vi "Pass.vi"(8 "error in (no error)":errorcluster, 11 "Constraint in":refnum<class "Constraint.lvclass">) -> (0 "error out":errorcluster, 3 "Constraint out":refnum<class "Constraint.lvclass">)   [LabVIEW 2017, in "Transparent Assertions.lvlib" / "Constraints.lvlib" / "Constraint.lvclass"]
doc: "Reports a successful test."
uses:
  Constraint.lvclass
  Frameworks/Test Framework/Test Framework.lvclass
  Frameworks/Test Framework Factory/Test Framework Factory.lvclass
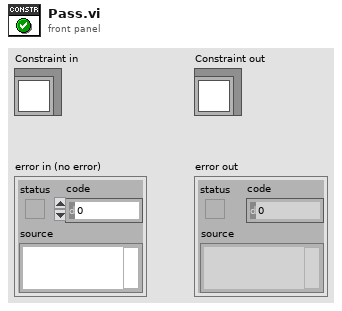
[diagram p1: front panel]
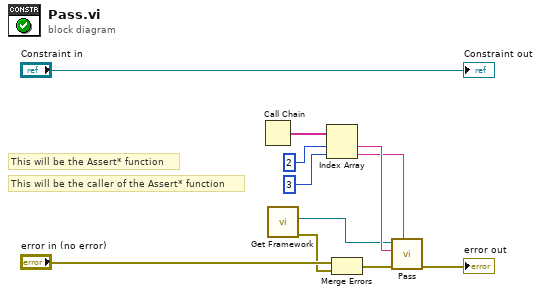
[diagram p0: block diagram]
diagram:
  # "This will be the Assert* function"
  # "This will be the caller of the Assert* function"
  n1 = Call Chain() -> (call chain=w8:string[])
  n2 = call "Get Framework.vi"() -> ("error out"=w1:errorcluster, "Test Framework"=w3:refnum<class "Test Framework.lvclass">)  [unwired: 10 in]
  n3 = Index Array(array=w8, index #1=2 ("index"), index #2=3 ("index")) -> (element #1=w5:string, element #2=w4:string)
  n4 = Merge Errors("error in (no error)", w1) -> (w2:errorcluster)
  n5 = call-dynamic "Pass.vi"("Caller"=w4, "error in (no error)"=w2, "Assertion"=w5, "Test Framework in"=w3) -> ("error out"=→"error out":errorcluster)  [unwired: 6 in, 1 out]
  "Constraint out" <- "Constraint in"
